vi "get Scaled Width And Height.vi"(11 "Texture in":refnum<class "Texture.lvclass">) -> (2 "Height":i32, 3 "Width":i32)   [LabVIEW 2021, in "Texture.lvclass"]
uses:
  Texture.lvclass
  Texture.lvclass/Texture.ctl
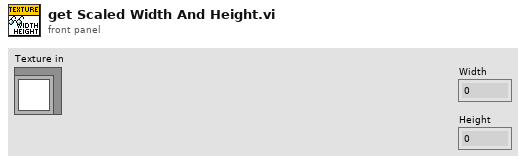
[diagram p1: front panel]
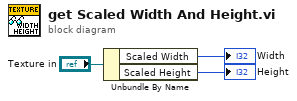
[diagram p0: block diagram]
diagram:
  n1 = Unbundle By Name("Texture in") -> ("Scaled Width"=→"Width":i32, "Scaled Height"=→"Height":i32)
